vi "MV3D RGBD Get Gig E Device List.vi"(10 "nMaxDeviceCount":u32) -> (0 "pDeviceCount out":u32, 1 "MV3D_RGBD_GigEDEVICE_ByteINFO out":T1(array[cluster]), 2 "MV3D_RGBD_GigEDEVICE_INFO out":T2(array[cluster]), 3 "function return":i32)   [LabVIEW 2015, in "Mv3dRgbdEx.lvlib"]
doc: "MV3D_RGBD_API_Ex MV3D_RGBD_STATUS MV3D_RGBD_GetGigEDeviceList(MV3D_RGBD_GigEDEVICE_INFO* pstGigEDeviceInfos, uint32_t nMaxDeviceCount, uint32_t* pDeviceCount);"
uses:
  <userlib>/Mv3dRgbdEx/Mv3dRgbdEx.lvlib
  <userlib>/Mv3dRgbdEx/Mv3dRgbdEx.dll
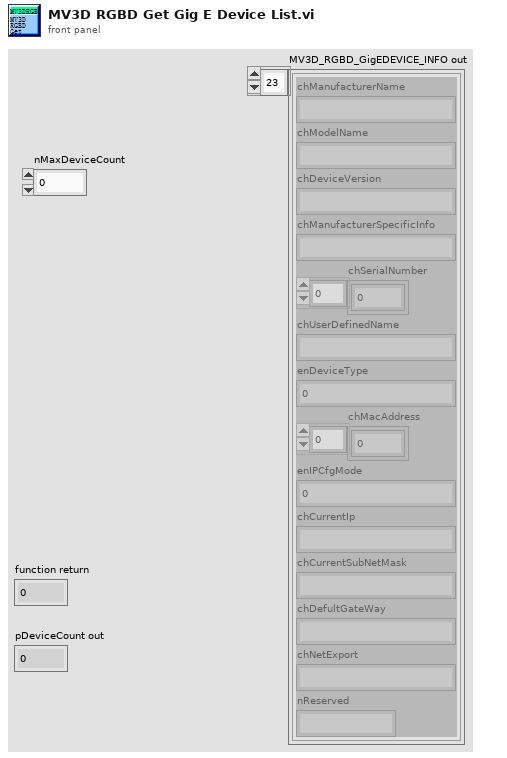
[diagram p1: front panel]
types:
  T1 = cluster{"chManufacturerName[0]":i8, "chManufacturerName[1]":i8, "chManufacturerName[2]":i8, "chManufacturerName[3]":i8, "chManufacturerName[4]":i8, "chManufacturerName[5]":i8, "chManufacturerName[6]":i8, "chManufacturerName[7]":i8, "chManufacturerName[8]":i8, "chManufacturerName[9]":i8, "chManufacturerName[10]":i8, "chManufacturerName[11]":i8, "chManufacturerName[12]":i8, "chManufacturerName[13]":i8, "chManufacturerName[14]":i8, "chManufacturerName[15]":i8, "chManufacturerName[16]":i8, "chManufacturerName[17]":i8, "chManufacturerName[18]":i8, "chManufacturerName[19]":i8, "chManufacturerName[20]":i8, "chManufacturerName[21]":i8, "chManufacturerName[22]":i8, "chManufacturerName[23]":i8, "chManufacturerName[24]":i8, "chManufacturerName[25]":i8, "chManufacturerName[26]":i8, "chManufacturerName[27]":i8, "chManufacturerName[28]":i8, "chManufacturerName[29]":i8, "chManufacturerName[30]":i8, "chManufacturerName[31]":i8, "chModelName[0]":i8, "chModelName[1]":i8, "chModelName[2]":i8, "chModelName[3]":i8, "chModelName[4]":i8, "chModelName[5]":i8, "chModelName[6]":i8, "chModelName[7]":i8, "chModelName[8]":i8, "chModelName[9]":i8, "chModelName[10]":i8, "chModelName[11]":i8, "chModelName[12]":i8, "chModelName[13]":i8, "chModelName[14]":i8, "chModelName[15]":i8, "chModelName[16]":i8, "chModelName[17]":i8, "chModelName[18]":i8, "chModelName[19]":i8, "chModelName[20]":i8, "chModelName[21]":i8, "chModelName[22]":i8, "chModelName[23]":i8, "chModelName[24]":i8, "chModelName[25]":i8, "chModelName[26]":i8, "chModelName[27]":i8, "chModelName[28]":i8, "chModelName[29]":i8, "chModelName[30]":i8, "chModelName[31]":i8, "chDeviceVersion[0]":i8, "chDeviceVersion[1]":i8, "chDeviceVersion[2]":i8, "chDeviceVersion[3]":i8, "chDeviceVersion[4]":i8, "chDeviceVersion[5]":i8, "chDeviceVersion[6]":i8, "chDeviceVersion[7]":i8, "chDeviceVersion[8]":i8, "chDeviceVersion[9]":i8, "chDeviceVersion[10]":i8, "chDeviceVersion[11]":i8, "chDeviceVersion[12]":i8, "chDeviceVersion[13]":i8, "chDeviceVersion[14]":i8, "chDeviceVersion[15]":i8, "chDeviceVersion[16]":i8, "chDeviceVersion[17]":i8, "chDeviceVersion[18]":i8, "chDeviceVersion[19]":i8, "chDeviceVersion[20]":i8, "chDeviceVersion[21]":i8, "chDeviceVersion[22]":i8, "chDeviceVersion[23]":i8, "chDeviceVersion[24]":i8, "chDeviceVersion[25]":i8, "chDeviceVersion[26]":i8, "chDeviceVersion[27]":i8, "chDeviceVersion[28]":i8, "chDeviceVersion[29]":i8, "chDeviceVersion[30]":i8, "chDeviceVersion[31]":i8, "chManufacturerSpecificInfo[0]":i8, "chManufacturerSpecificInfo[1]":i8, "chManufacturerSpecificInfo[2]":i8, "chManufacturerSpecificInfo[3]":i8, "chManufacturerSpecificInfo[4]":i8, "chManufacturerSpecificInfo[5]":i8, "chManufacturerSpecificInfo[6]":i8, "chManufacturerSpecificInfo[7]":i8, "chManufacturerSpecificInfo[8]":i8, "chManufacturerSpecificInfo[9]":i8, "chManufacturerSpecificInfo[10]":i8, "chManufacturerSpecificInfo[11]":i8, "chManufacturerSpecificInfo[12]":i8, "chManufacturerSpecificInfo[13]":i8, "chManufacturerSpecificInfo[14]":i8, "chManufacturerSpecificInfo[15]":i8, "chManufacturerSpecificInfo[16]":i8, "chManufacturerSpecificInfo[17]":i8, "chManufacturerSpecificInfo[18]":i8, "chManufacturerSpecificInfo[19]":i8, "chManufacturerSpecificInfo[20]":i8, "chManufacturerSpecificInfo[21]":i8, "chManufacturerSpecificInfo[22]":i8, "chManufacturerSpecificInfo[23]":i8, "chManufacturerSpecificInfo[24]":i8, "chManufacturerSpecificInfo[25]":i8, "chManufacturerSpecificInfo[26]":i8, "chManufacturerSpecificInfo[27]":i8, "chManufacturerSpecificInfo[28]":i8, "chManufacturerSpecificInfo[29]":i8, "chManufacturerSpecificInfo[30]":i8, "chManufacturerSpecificInfo[31]":i8, "chManufacturerSpecificInfo[32]":i8, "chManufacturerSpecificInfo[33]":i8, "chManufacturerSpecificInfo[34]":i8, "chManufacturerSpecificInfo[35]":i8, "chManufacturerSpecificInfo[36]":i8, "chManufacturerSpecificInfo[37]":i8, "chManufacturerSpecificInfo[38]":i8, "chManufacturerSpecificInfo[39]":i8, "chManufacturerSpecificInfo[40]":i8, "chManufacturerSpecificInfo[41]":i8, "chManufacturerSpecificInfo[42]":i8, "chManufacturerSpecificInfo[43]":i8, "chManufacturerSpecificInfo[44]":i8, "chManufacturerSpecificInfo[45]":i8, "chManufacturerSpecificInfo[46]":i8, "chManufacturerSpecificInfo[47]":i8, "chSerialNumber[0]":i8, "chSerialNumber[1]":i8, "chSerialNumber[2]":i8, "chSerialNumber[3]":i8, "chSerialNumber[4]":i8, "chSerialNumber[5]":i8, "chSerialNumber[6]":i8, "chSerialNumber[7]":i8, "chSerialNumber[8]":i8, "chSerialNumber[9]":i8, "chSerialNumber[10]":i8, "chSerialNumber[11]":i8, "chSerialNumber[12]":i8, "chSerialNumber[13]":i8, "chSerialNumber[14]":i8, "chSerialNumber[15]":i8, "chUserDefinedName[0]":i8, "chUserDefinedName[1]":i8, "chUserDefinedName[2]":i8, "chUserDefinedName[3]":i8, "chUserDefinedName[4]":i8, "chUserDefinedName[5]":i8, "chUserDefinedName[6]":i8, "chUserDefinedName[7]":i8, "chUserDefinedName[8]":i8, "chUserDefinedName[9]":i8, "chUserDefinedName[10]":i8, "chUserDefinedName[11]":i8, "chUserDefinedName[12]":i8, "chUserDefinedName[13]":i8, "chUserDefinedName[14]":i8, "chUserDefinedName[15]":i8, "enDeviceType":i32, "chMacAddress[0]":u8, "chMacAddress[1]":u8, "chMacAddress[2]":u8, "chMacAddress[3]":u8, "chMacAddress[4]":u8, "chMacAddress[5]":u8, "chMacAddress[6]":u8, "chMacAddress[7]":u8, "enIPCfgMode":i32, "chCurrentIp[0]":i8, "chCurrentIp[1]":i8, "chCurrentIp[2]":i8, "chCurrentIp[3]":i8, "chCurrentIp[4]":i8, "chCurrentIp[5]":i8, "chCurrentIp[6]":i8, "chCurrentIp[7]":i8, "chCurrentIp[8]":i8, "chCurrentIp[9]":i8, "chCurrentIp[10]":i8, "chCurrentIp[11]":i8, "chCurrentIp[12]":i8, "chCurrentIp[13]":i8, "chCurrentIp[14]":i8, "chCurrentIp[15]":i8, "chCurrentSubNetMask[0]":i8, "chCurrentSubNetMask[1]":i8, "chCurrentSubNetMask[2]":i8, "chCurrentSubNetMask[3]":i8, "chCurrentSubNetMask[4]":i8, "chCurrentSubNetMask[5]":i8, "chCurrentSubNetMask[6]":i8, "chCurrentSubNetMask[7]":i8, "chCurrentSubNetMask[8]":i8, "chCurrentSubNetMask[9]":i8, "chCurrentSubNetMask[10]":i8, "chCurrentSubNetMask[11]":i8, "chCurrentSubNetMask[12]":i8, "chCurrentSubNetMask[13]":i8, "chCurrentSubNetMask[14]":i8, "chCurrentSubNetMask[15]":i8, "chDefultGateWay[0]":i8, "chDefultGateWay[1]":i8, "chDefultGateWay[2]":i8, "chDefultGateWay[3]":i8, "chDefultGateWay[4]":i8, "chDefultGateWay[5]":i8, "chDefultGateWay[6]":i8, "chDefultGateWay[7]":i8, "chDefultGateWay[8]":i8, "chDefultGateWay[9]":i8, "chDefultGateWay[10]":i8, "chDefultGateWay[11]":i8, "chDefultGateWay[12]":i8, "chDefultGateWay[13]":i8, "chDefultGateWay[14]":i8, "chDefultGateWay[15]":i8, "chNetExport[0]":i8, "chNetExport[1]":i8, "chNetExport[2]":i8, "chNetExport[3]":i8, "chNetExport[4]":i8, "chNetExport[5]":i8, "chNetExport[6]":i8, "chNetExport[7]":i8, "chNetExport[8]":i8, "chNetExport[9]":i8, "chNetExport[10]":i8, "chNetExport[11]":i8, "chNetExport[12]":i8, "chNetExport[13]":i8, "chNetExport[14]":i8, "chNetExport[15]":i8, "nReserved[0]":u8, "nReserved[1]":u8, "nReserved[2]":u8, "nReserved[3]":u8, "nReserved[4]":u8, "nReserved[5]":u8, "nReserved[6]":u8, "nReserved[7]":u8, "nReserved[8]":u8, "nReserved[9]":u8, "nReserved[10]":u8, "nReserved[11]":u8, "nReserved[12]":u8, "nReserved[13]":u8, "nReserved[14]":u8, "nReserved[15]":u8}[]
  T2 = cluster{"chManufacturerName":string, "chModelName":string, "chDeviceVersion":string, "chManufacturerSpecificInfo":string, "chSerialNumber":u8[], "chUserDefinedName":string, "enDeviceType":i32, "chMacAddress":u8[], "enIPCfgMode":i32, "chCurrentIp":string, "chCurrentSubNetMask":string, "chDefultGateWay":string, "chNetExport":string, "nReserved":string}[]
  T3 = cluster{"chManufacturerName[0]":i8, "chManufacturerName[1]":i8, "chManufacturerName[2]":i8, "chManufacturerName[3]":i8, "chManufacturerName[4]":i8, "chManufacturerName[5]":i8, "chManufacturerName[6]":i8, "chManufacturerName[7]":i8, "chManufacturerName[8]":i8, "chManufacturerName[9]":i8, "chManufacturerName[10]":i8, "chManufacturerName[11]":i8, "chManufacturerName[12]":i8, "chManufacturerName[13]":i8, "chManufacturerName[14]":i8, "chManufacturerName[15]":i8, "chManufacturerName[16]":i8, "chManufacturerName[17]":i8, "chManufacturerName[18]":i8, "chManufacturerName[19]":i8, "chManufacturerName[20]":i8, "chManufacturerName[21]":i8, "chManufacturerName[22]":i8, "chManufacturerName[23]":i8, "chManufacturerName[24]":i8, "chManufacturerName[25]":i8, "chManufacturerName[26]":i8, "chManufacturerName[27]":i8, "chManufacturerName[28]":i8, "chManufacturerName[29]":i8, "chManufacturerName[30]":i8, "chManufacturerName[31]":i8, "chModelName[0]":i8, "chModelName[1]":i8, "chModelName[2]":i8, "chModelName[3]":i8, "chModelName[4]":i8, "chModelName[5]":i8, "chModelName[6]":i8, "chModelName[7]":i8, "chModelName[8]":i8, "chModelName[9]":i8, "chModelName[10]":i8, "chModelName[11]":i8, "chModelName[12]":i8, "chModelName[13]":i8, "chModelName[14]":i8, "chModelName[15]":i8, "chModelName[16]":i8, "chModelName[17]":i8, "chModelName[18]":i8, "chModelName[19]":i8, "chModelName[20]":i8, "chModelName[21]":i8, "chModelName[22]":i8, "chModelName[23]":i8, "chModelName[24]":i8, "chModelName[25]":i8, "chModelName[26]":i8, "chModelName[27]":i8, "chModelName[28]":i8, "chModelName[29]":i8, "chModelName[30]":i8, "chModelName[31]":i8, "chDeviceVersion[0]":i8, "chDeviceVersion[1]":i8, "chDeviceVersion[2]":i8, "chDeviceVersion[3]":i8, "chDeviceVersion[4]":i8, "chDeviceVersion[5]":i8, "chDeviceVersion[6]":i8, "chDeviceVersion[7]":i8, "chDeviceVersion[8]":i8, "chDeviceVersion[9]":i8, "chDeviceVersion[10]":i8, "chDeviceVersion[11]":i8, "chDeviceVersion[12]":i8, "chDeviceVersion[13]":i8, "chDeviceVersion[14]":i8, "chDeviceVersion[15]":i8, "chDeviceVersion[16]":i8, "chDeviceVersion[17]":i8, "chDeviceVersion[18]":i8, "chDeviceVersion[19]":i8, "chDeviceVersion[20]":i8, "chDeviceVersion[21]":i8, "chDeviceVersion[22]":i8, "chDeviceVersion[23]":i8, "chDeviceVersion[24]":i8, "chDeviceVersion[25]":i8, "chDeviceVersion[26]":i8, "chDeviceVersion[27]":i8, "chDeviceVersion[28]":i8, "chDeviceVersion[29]":i8, "chDeviceVersion[30]":i8, "chDeviceVersion[31]":i8, "chManufacturerSpecificInfo[0]":i8, "chManufacturerSpecificInfo[1]":i8, "chManufacturerSpecificInfo[2]":i8, "chManufacturerSpecificInfo[3]":i8, "chManufacturerSpecificInfo[4]":i8, "chManufacturerSpecificInfo[5]":i8, "chManufacturerSpecificInfo[6]":i8, "chManufacturerSpecificInfo[7]":i8, "chManufacturerSpecificInfo[8]":i8, "chManufacturerSpecificInfo[9]":i8, "chManufacturerSpecificInfo[10]":i8, "chManufacturerSpecificInfo[11]":i8, "chManufacturerSpecificInfo[12]":i8, "chManufacturerSpecificInfo[13]":i8, "chManufacturerSpecificInfo[14]":i8, "chManufacturerSpecificInfo[15]":i8, "chManufacturerSpecificInfo[16]":i8, "chManufacturerSpecificInfo[17]":i8, "chManufacturerSpecificInfo[18]":i8, "chManufacturerSpecificInfo[19]":i8, "chManufacturerSpecificInfo[20]":i8, "chManufacturerSpecificInfo[21]":i8, "chManufacturerSpecificInfo[22]":i8, "chManufacturerSpecificInfo[23]":i8, "chManufacturerSpecificInfo[24]":i8, "chManufacturerSpecificInfo[25]":i8, "chManufacturerSpecificInfo[26]":i8, "chManufacturerSpecificInfo[27]":i8, "chManufacturerSpecificInfo[28]":i8, "chManufacturerSpecificInfo[29]":i8, "chManufacturerSpecificInfo[30]":i8, "chManufacturerSpecificInfo[31]":i8, "chManufacturerSpecificInfo[32]":i8, "chManufacturerSpecificInfo[33]":i8, "chManufacturerSpecificInfo[34]":i8, "chManufacturerSpecificInfo[35]":i8, "chManufacturerSpecificInfo[36]":i8, "chManufacturerSpecificInfo[37]":i8, "chManufacturerSpecificInfo[38]":i8, "chManufacturerSpecificInfo[39]":i8, "chManufacturerSpecificInfo[40]":i8, "chManufacturerSpecificInfo[41]":i8, "chManufacturerSpecificInfo[42]":i8, "chManufacturerSpecificInfo[43]":i8, "chManufacturerSpecificInfo[44]":i8, "chManufacturerSpecificInfo[45]":i8, "chManufacturerSpecificInfo[46]":i8, "chManufacturerSpecificInfo[47]":i8, "chSerialNumber[0]":i8, "chSerialNumber[1]":i8, "chSerialNumber[2]":i8, "chSerialNumber[3]":i8, "chSerialNumber[4]":i8, "chSerialNumber[5]":i8, "chSerialNumber[6]":i8, "chSerialNumber[7]":i8, "chSerialNumber[8]":i8, "chSerialNumber[9]":i8, "chSerialNumber[10]":i8, "chSerialNumber[11]":i8, "chSerialNumber[12]":i8, "chSerialNumber[13]":i8, "chSerialNumber[14]":i8, "chSerialNumber[15]":i8, "chUserDefinedName[0]":i8, "chUserDefinedName[1]":i8, "chUserDefinedName[2]":i8, "chUserDefinedName[3]":i8, "chUserDefinedName[4]":i8, "chUserDefinedName[5]":i8, "chUserDefinedName[6]":i8, "chUserDefinedName[7]":i8, "chUserDefinedName[8]":i8, "chUserDefinedName[9]":i8, "chUserDefinedName[10]":i8, "chUserDefinedName[11]":i8, "chUserDefinedName[12]":i8, "chUserDefinedName[13]":i8, "chUserDefinedName[14]":i8, "chUserDefinedName[15]":i8, "enDeviceType":i32, "chMacAddress[0]":u8, "chMacAddress[1]":u8, "chMacAddress[2]":u8, "chMacAddress[3]":u8, "chMacAddress[4]":u8, "chMacAddress[5]":u8, "chMacAddress[6]":u8, "chMacAddress[7]":u8, "enIPCfgMode":i32, "chCurrentIp[0]":i8, "chCurrentIp[1]":i8, "chCurrentIp[2]":i8, "chCurrentIp[3]":i8, "chCurrentIp[4]":i8, "chCurrentIp[5]":i8, "chCurrentIp[6]":i8, "chCurrentIp[7]":i8, "chCurrentIp[8]":i8, "chCurrentIp[9]":i8, "chCurrentIp[10]":i8, "chCurrentIp[11]":i8, "chCurrentIp[12]":i8, "chCurrentIp[13]":i8, "chCurrentIp[14]":i8, "chCurrentIp[15]":i8, "chCurrentSubNetMask[0]":i8, "chCurrentSubNetMask[1]":i8, "chCurrentSubNetMask[2]":i8, "chCurrentSubNetMask[3]":i8, "chCurrentSubNetMask[4]":i8, "chCurrentSubNetMask[5]":i8, "chCurrentSubNetMask[6]":i8, "chCurrentSubNetMask[7]":i8, "chCurrentSubNetMask[8]":i8, "chCurrentSubNetMask[9]":i8, "chCurrentSubNetMask[10]":i8, "chCurrentSubNetMask[11]":i8, "chCurrentSubNetMask[12]":i8, "chCurrentSubNetMask[13]":i8, "chCurrentSubNetMask[14]":i8, "chCurrentSubNetMask[15]":i8, "chDefultGateWay[0]":i8, "chDefultGateWay[1]":i8, "chDefultGateWay[2]":i8, "chDefultGateWay[3]":i8, "chDefultGateWay[4]":i8, "chDefultGateWay[5]":i8, "chDefultGateWay[6]":i8, "chDefultGateWay[7]":i8, "chDefultGateWay[8]":i8, "chDefultGateWay[9]":i8, "chDefultGateWay[10]":i8, "chDefultGateWay[11]":i8, "chDefultGateWay[12]":i8, "chDefultGateWay[13]":i8, "chDefultGateWay[14]":i8, "chDefultGateWay[15]":i8, "chNetExport[0]":i8, "chNetExport[1]":i8, "chNetExport[2]":i8, "chNetExport[3]":i8, "chNetExport[4]":i8, "chNetExport[5]":i8, "chNetExport[6]":i8, "chNetExport[7]":i8, "chNetExport[8]":i8, "chNetExport[9]":i8, "chNetExport[10]":i8, "chNetExport[11]":i8, "chNetExport[12]":i8, "chNetExport[13]":i8, "chNetExport[14]":i8, "chNetExport[15]":i8, "nReserved[0]":u8, "nReserved[1]":u8, "nReserved[2]":u8, "nReserved[3]":u8, "nReserved[4]":u8, "nReserved[5]":u8, "nReserved[6]":u8, "nReserved[7]":u8, "nReserved[8]":u8, "nReserved[9]":u8, "nReserved[10]":u8, "nReserved[11]":u8, "nReserved[12]":u8, "nReserved[13]":u8, "nReserved[14]":u8, "nReserved[15]":u8}
  T4 = cluster{"chManufacturerName":string, "chModelName":string, "chDeviceVersion":string, "chManufacturerSpecificInfo":string, "chSerialNumber":u8[], "chUserDefinedName":string, "enDeviceType":i32, "chMacAddress":u8[], "enIPCfgMode":i32, "chCurrentIp":string, "chCurrentSubNetMask":string, "chDefultGateWay":string, "chNetExport":string, "nReserved":string}
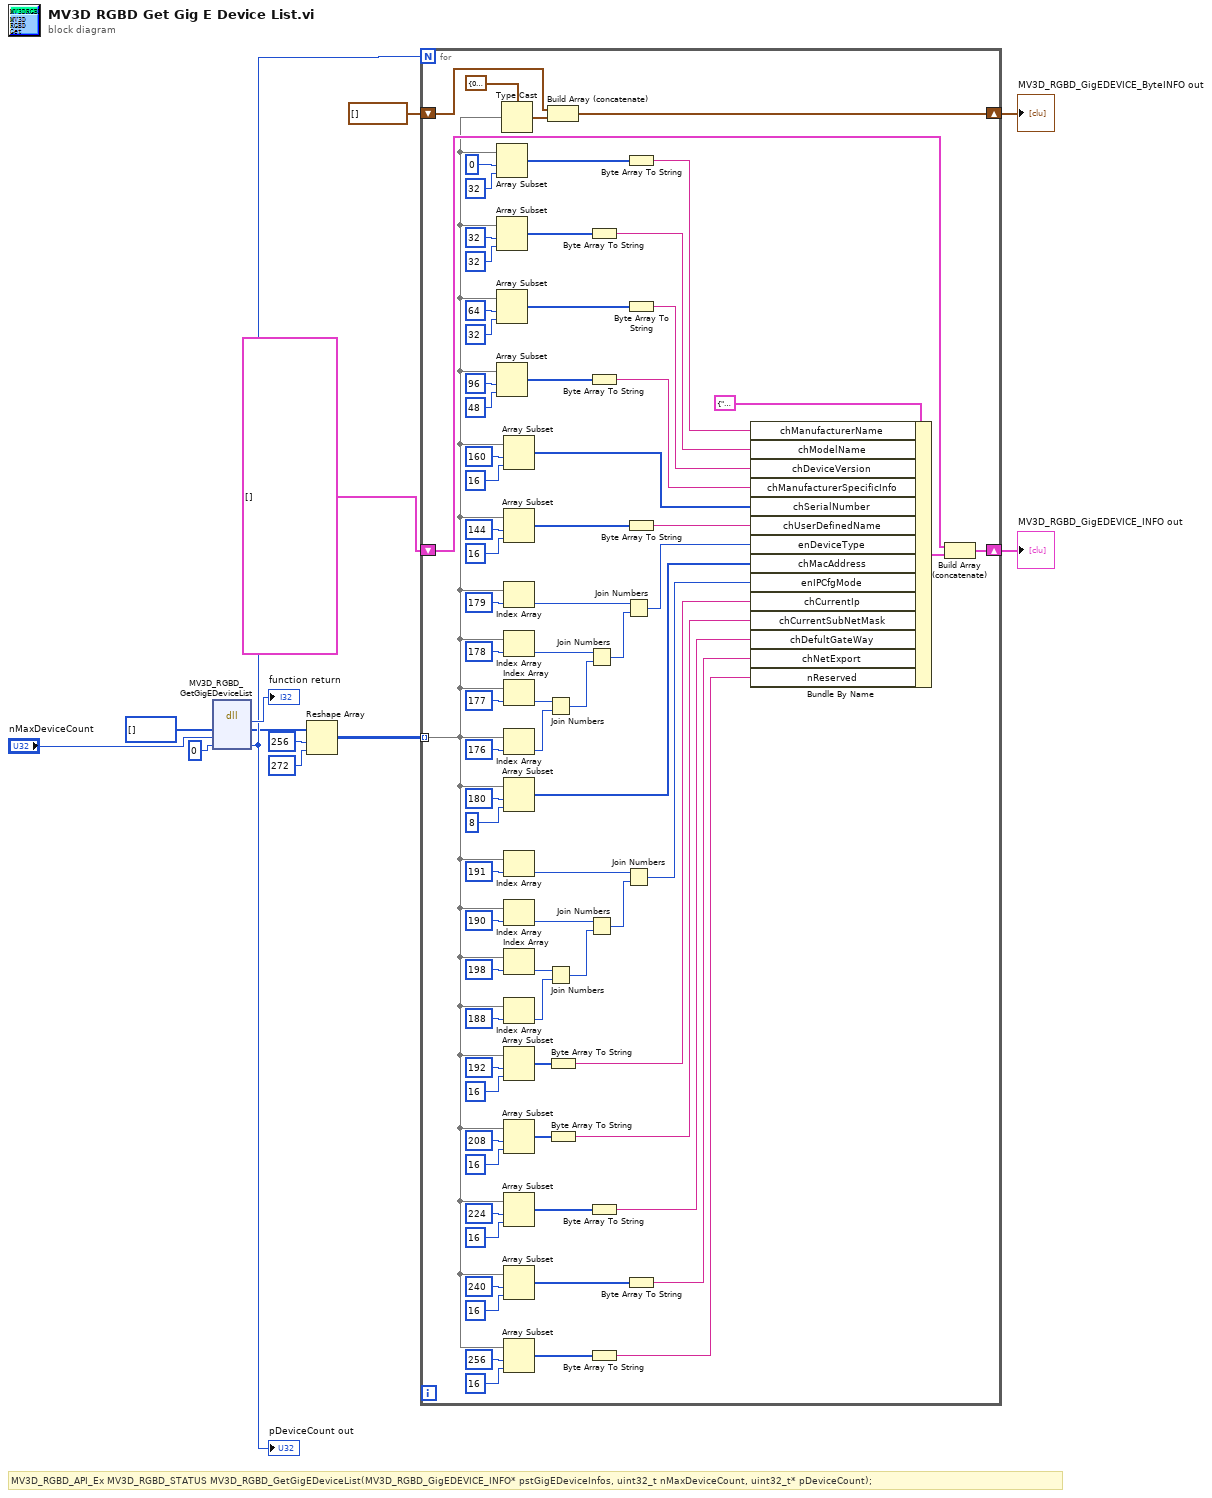
[diagram p0: block diagram]
diagram:
  # "MV3D_RGBD_API_Ex MV3D_RGBD_STATUS MV3D_RGBD_GetGigEDeviceList(MV3D_RGBD_GigEDEVICE_INFO* pstGigEDeviceInfos, uint32_t nMaxDeviceCount, uint32_t* pDeviceCount);"
  n1 = dll-call lib="C:/Program Files (x86)/National Instruments/LabVIEW 2015/user.lib/Mv3dRgbdEx/Mv3dRgbdEx.*" fn="MV3D_RGBD_GetGigEDeviceList"("pstGigEDeviceInfos"=u8[] [] ("pstGigEDeviceInfos 4"), "nMaxDeviceCount"="nMaxDeviceCount", "pDeviceCount"=u32 0) -> ("返回类型"=→"function return":i32, "pstGigEDeviceInfos"=w8:u8[], "pDeviceCount"=w9:u32)  [unwired: 4 in, 2 out]
  "pDeviceCount out" <- w9
  n2 = Reshape Array(w8, 256 ("维数大小"), 272 ("维数大小")) -> (w5:u8[][])
  n3 = for {
    N: w9 -> [_]
    shift-right: [w46] -> w3
    shift-left: T2 [] -> [w19]
    tunnel: w5 -> [w17] mode=indexing
    shift-right: [w16] -> w2
    shift-left: T1 [] ("*(类型 *) &x") -> [w14]
    n4 = Array Subset(array=w17, index=0 ("索引"), length=32 ("长度")) -> (w88:u8[])
    n5 = Array Subset(array=w17, index=32 ("索引"), length=32 ("长度")) -> (w85:u8[])
    n6 = Array Subset(array=w17, index=64 ("索引"), length=32 ("长度")) -> (w78:u8[])
    n7 = Array Subset(array=w17, index=96 ("索引"), length=48 ("长度")) -> (w82:u8[])
    n8 = Type Cast(type=T3 {"chManufacturerName[0]"=0, "chManufacturerName[1]"=0, "chManufacturerName[2]"=0, "chManufacturerName[3]"=0, "chManufacturerName[4]"=0, "chManufacturerName[5]"=0, "chManufacturerName[6]"=0, "chManufacturerName[7]"=0, "chManufacturerName[8]"=0, "chManufacturerName[9]"=0, "chManufacturerName[10]"=0, "chManufacturerName[11]"=0, "chManufacturerName[12]"=0, "chManufacturerName[13]"=0, "chManufacturerName[14]"=0, "chManufacturerName[15]"=0, "chManufacturerName[16]"=0, "chManufacturerName[17]"=0, "chManufacturerName[18]"=0, "chManufacturerName[19]"=0, "chManufacturerName[20]"=0, "chManufacturerName[21]"=0, "chManufacturerName[22]"=0, "chManufacturerName[23]"=0, "chManufacturerName[24]"=0, "chManufacturerName[25]"=0, "chManufacturerName[26]"=0, "chManufacturerName[27]"=0, "chManufacturerName[28]"=0, "chManufacturerName[29]"=0, "chManufacturerName[30]"=0, "chManufacturerName[31]"=0, "chModelName[0]"=0, "chModelName[1]"=0, "chModelName[2]"=0, "chModelName[3]"=0, "chModelName[4]"=0, "chModelName[5]"=0, "chModelName[6]"=0, "chModelName[7]"=0, "chModelName[8]"=0, "chModelName[9]"=0, "chModelName[10]"=0, "chModelName[11]"=0, "chModelName[12]"=0, "chModelName[13]"=0, "chModelName[14]"=0, "chModelName[15]"=0, "chModelName[16]"=0, "chModelName[17]"=0, "chModelName[18]"=0, "chModelName[19]"=0, "chModelName[20]"=0, "chModelName[21]"=0, "chModelName[22]"=0, "chModelName[23]"=0, "chModelName[24]"=0, "chModelName[25]"=0, "chModelName[26]"=0, "chModelName[27]"=0, "chModelName[28]"=0, "chModelName[29]"=0, "chModelName[30]"=0, "chModelName[31]"=0, "chDeviceVersion[0]"=0, "chDeviceVersion[1]"=0, "chDeviceVersion[2]"=0, "chDeviceVersion[3]"=0, "chDeviceVersion[4]"=0, "chDeviceVersion[5]"=0, "chDeviceVersion[6]"=0, "chDeviceVersion[7]"=0, "chDeviceVersion[8]"=0, "chDeviceVersion[9]"=0, "chDeviceVersion[10]"=0, "chDeviceVersion[11]"=0, "chDeviceVersion[12]"=0, "chDeviceVersion[13]"=0, "chDeviceVersion[14]"=0, "chDeviceVersion[15]"=0, "chDeviceVersion[16]"=0, "chDeviceVersion[17]"=0, "chDeviceVersion[18]"=0, "chDeviceVersion[19]"=0, "chDeviceVersion[20]"=0, "chDeviceVersion[21]"=0, "chDeviceVersion[22]"=0, "chDeviceVersion[23]"=0, "chDeviceVersion[24]"=0, "chDeviceVersion[25]"=0, "chDeviceVersion[26]"=0, "chDeviceVersion[27]"=0, "chDeviceVersion[28]"=0, "chDeviceVersion[29]"=0, "chDeviceVersion[30]"=0, "chDeviceVersion[31]"=0, "chManufacturerSpecificInfo[0]"=0, "chManufacturerSpecificInfo[1]"=0, "chManufacturerSpecificInfo[2]"=0, "chManufacturerSpecificInfo[3]"=0, "chManufacturerSpecificInfo[4]"=0, "chManufacturerSpecificInfo[5]"=0, "chManufacturerSpecificInfo[6]"=0, "chManufacturerSpecificInfo[7]"=0, "chManufacturerSpecificInfo[8]"=0, "chManufacturerSpecificInfo[9]"=0, "chManufacturerSpecificInfo[10]"=0, "chManufacturerSpecificInfo[11]"=0, "chManufacturerSpecificInfo[12]"=0, "chManufacturerSpecificInfo[13]"=0, "chManufacturerSpecificInfo[14]"=0, "chManufacturerSpecificInfo[15]"=0, "chManufacturerSpecificInfo[16]"=0, "chManufacturerSpecificInfo[17]"=0, "chManufacturerSpecificInfo[18]"=0, "chManufacturerSpecificInfo[19]"=0, "chManufacturerSpecificInfo[20]"=0, "chManufacturerSpecificInfo[21]"=0, "chManufacturerSpecificInfo[22]"=0, "chManufacturerSpecificInfo[23]"=0, "chManufacturerSpecificInfo[24]"=0, "chManufacturerSpecificInfo[25]"=0, "chManufacturerSpecificInfo[26]"=0, "chManufacturerSpecificInfo[27]"=0, "chManufacturerSpecificInfo[28]"=0, "chManufacturerSpecificInfo[29]"=0, "chManufacturerSpecificInfo[30]"=0, "chManufacturerSpecificInfo[31]"=0, "chManufacturerSpecificInfo[32]"=0, "chManufacturerSpecificInfo[33]"=0, "chManufacturerSpecificInfo[34]"=0, "chManufacturerSpecificInfo[35]"=0, "chManufacturerSpecificInfo[36]"=0, "chManufacturerSpecificInfo[37]"=0, "chManufacturerSpecificInfo[38]"=0, "chManufacturerSpecificInfo[39]"=0, "chManufacturerSpecificInfo[40]"=0, "chManufacturerSpecificInfo[41]"=0, "chManufacturerSpecificInfo[42]"=0, "chManufacturerSpecificInfo[43]"=0, "chManufacturerSpecificInfo[44]"=0, "chManufacturerSpecificInfo[45]"=0, "chManufacturerSpecificInfo[46]"=0, "chManufacturerSpecificInfo[47]"=0, "chSerialNumber[0]"=0, "chSerialNumber[1]"=0, "chSerialNumber[2]"=0, "chSerialNumber[3]"=0, "chSerialNumber[4]"=0, "chSerialNumber[5]"=0, "chSerialNumber[6]"=0, "chSerialNumber[7]"=0, "chSerialNumber[8]"=0, "chSerialNumber[9]"=0, "chSerialNumber[10]"=0, "chSerialNumber[11]"=0, "chSerialNumber[12]"=0, "chSerialNumber[13]"=0, "chSerialNumber[14]"=0, "chSerialNumber[15]"=0, "chUserDefinedName[0]"=0, "chUserDefinedName[1]"=0, "chUserDefinedName[2]"=0, "chUserDefinedName[3]"=0, "chUserDefinedName[4]"=0, "chUserDefinedName[5]"=0, "chUserDefinedName[6]"=0, "chUserDefinedName[7]"=0, "chUserDefinedName[8]"=0, "chUserDefinedName[9]"=0, "chUserDefinedName[10]"=0, "chUserDefinedName[11]"=0, "chUserDefinedName[12]"=0, "chUserDefinedName[13]"=0, "chUserDefinedName[14]"=0, "chUserDefinedName[15]"=0, "enDeviceType"=0, "chMacAddress[0]"=0, "chMacAddress[1]"=0, "chMacAddress[2]"=0, "chMacAddress[3]"=0, "chMacAddress[4]"=0, "chMacAddress[5]"=0, "chMacAddress[6]"=0, "chMacAddress[7]"=0, "enIPCfgMode"=0, "chCurrentIp[0]"=0, "chCurrentIp[1]"=0, "chCurrentIp[2]"=0, "chCurrentIp[3]"=0, "chCurrentIp[4]"=0, "chCurrentIp[5]"=0, "chCurrentIp[6]"=0, "chCurrentIp[7]"=0, "chCurrentIp[8]"=0, "chCurrentIp[9]"=0, "chCurrentIp[10]"=0, "chCurrentIp[11]"=0, "chCurrentIp[12]"=0, "chCurrentIp[13]"=0, "chCurrentIp[14]"=0, "chCurrentIp[15]"=0, "chCurrentSubNetMask[0]"=0, "chCurrentSubNetMask[1]"=0, "chCurrentSubNetMask[2]"=0, "chCurrentSubNetMask[3]"=0, "chCurrentSubNetMask[4]"=0, "chCurrentSubNetMask[5]"=0, "chCurrentSubNetMask[6]"=0, "chCurrentSubNetMask[7]"=0, "chCurrentSubNetMask[8]"=0, "chCurrentSubNetMask[9]"=0, "chCurrentSubNetMask[10]"=0, "chCurrentSubNetMask[11]"=0, "chCurrentSubNetMask[12]"=0, "chCurrentSubNetMask[13]"=0, "chCurrentSubNetMask[14]"=0, "chCurrentSubNetMask[15]"=0, "chDefultGateWay[0]"=0, "chDefultGateWay[1]"=0, "chDefultGateWay[2]"=0, "chDefultGateWay[3]"=0, "chDefultGateWay[4]"=0, "chDefultGateWay[5]"=0, "chDefultGateWay[6]"=0, "chDefultGateWay[7]"=0, "chDefultGateWay[8]"=0, "chDefultGateWay[9]"=0, "chDefultGateWay[10]"=0, "chDefultGateWay[11]"=0, "chDefultGateWay[12]"=0, "chDefultGateWay[13]"=0, "chDefultGateWay[14]"=0, "chDefultGateWay[15]"=0, "chNetExport[0]"=0, "chNetExport[1]"=0, "chNetExport[2]"=0, "chNetExport[3]"=0, "chNetExport[4]"=0, "chNetExport[5]"=0, "chNetExport[6]"=0, "chNetExport[7]"=0, "chNetExport[8]"=0, "chNetExport[9]"=0, "chNetExport[10]"=0, "chNetExport[11]"=0, "chNetExport[12]"=0, "chNetExport[13]"=0, "chNetExport[14]"=0, "chNetExport[15]"=0, "nReserved[0]"=0, "nReserved[1]"=0, "nReserved[2]"=0, "nReserved[3]"=0, "nReserved[4]"=0, "nReserved[5]"=0, "nReserved[6]"=0, "nReserved[7]"=0, "nReserved[8]"=0, "nReserved[9]"=0, "nReserved[10]"=0, "nReserved[11]"=0, "nReserved[12]"=0, "nReserved[13]"=0, "nReserved[14]"=0, "nReserved[15]"=0} ("pstGigeDeviceInfo out"), x=w17) -> (*(type *) &x=w15:T3)
    n9 = Array Subset(array=w17, index=160 ("索引"), length=16 ("长度")) -> (w28:u8[])
    n10 = Array Subset(array=w17, index=144 ("索引"), length=16 ("长度")) -> (w79:u8[])
    n11 = Index Array(array=w17, index=179 ("索引")) -> (element=w21:u8)
    n12 = Index Array(array=w17, index=178 ("索引")) -> (element=w22:u8)
    n13 = Index Array(array=w17, index=177 ("索引")) -> (element=w24:u8)
    n14 = Index Array(array=w17, index=176 ("索引")) -> (element=w25:u8)
    n15 = Array Subset(array=w17, index=180 ("索引"), length=8 ("长度")) -> (w26:u8[])
    n16 = Index Array(array=w17, index=191 ("索引")) -> (element=w39:u8)
    n17 = Index Array(array=w17, index=190 ("索引")) -> (element=w37:u8)
    n18 = Index Array(array=w17, index=198 ("索引")) -> (element=w35:u8)
    n19 = Index Array(array=w17, index=188 ("索引")) -> (element=w30:u8)
    n20 = Array Subset(array=w17, index=192 ("索引"), length=16 ("长度")) -> (w72:u8[])
    n21 = Array Subset(array=w17, index=208 ("索引"), length=16 ("长度")) -> (w70:u8[])
    n22 = Array Subset(array=w17, index=224 ("索引"), length=16 ("长度")) -> (w68:u8[])
    n23 = Array Subset(array=w17, index=240 ("索引"), length=16 ("长度")) -> (w66:u8[])
    n24 = Array Subset(array=w17, index=256 ("索引"), length=16 ("长度")) -> (w64:u8[])
    n25 = Join Numbers(hi=w24, lo=w25) -> ((hi.lo)=w23:u16)
    n26 = Join Numbers(hi=w35, lo=w30) -> ((hi.lo)=w34:u16)
    n27 = Build Array (concatenate)(w14, w15) -> (w16:T1)
    n28 = Byte Array To String(unsigned byte array=w72) -> (string=w51:string)
    n29 = Byte Array To String(unsigned byte array=w70) -> (string=w50:string)
    n30 = Join Numbers(hi=w22, lo=w23) -> ((hi.lo)=w20:u32)
    n31 = Join Numbers(hi=w37, lo=w34) -> ((hi.lo)=w33:u32)
    n32 = Byte Array To String(unsigned byte array=w85) -> (string=w55:string)
    n33 = Byte Array To String(unsigned byte array=w82) -> (string=w53:string)
    n34 = Byte Array To String(unsigned byte array=w68) -> (string=w49:string)
    n35 = Byte Array To String(unsigned byte array=w64) -> (string=w47:string)
    n36 = Join Numbers(hi=w21, lo=w20) -> ((hi.lo)=w41:u64)
    n37 = Join Numbers(hi=w39, lo=w33) -> ((hi.lo)=w32:u64)
    n38 = Byte Array To String(unsigned byte array=w88) -> (string=w56:string)
    n39 = Byte Array To String(unsigned byte array=w78) -> (string=w54:string)
    n40 = Byte Array To String(unsigned byte array=w79) -> (string=w52:string)
    n41 = Byte Array To String(unsigned byte array=w66) -> (string=w48:string)
    n42 = Bundle By Name(cluster=T4 {"chManufacturerName"="Hikrobot\u0000\u0000\u0000\u0000\u0000\u0000\u0000\u0000\u0000\u0000\u0000\u0000\u0000\u0000\u0000\u0000\u0000\u0000\u0000\u0000\u0000\u0000\u0000\u0000", "chModelName"="MV-DP2307-01H\u0000\u0000\u0000\u0000\u0000\u0000\u0000\u0000\u0000\u0000\u0000\u0000\u0000\u0000\u0000\u0000\u0000\u0000\u0000", "chDeviceVersion"="V1.2.1 220326 783627\u0000\u0000\u0000\u0000\u0000\u0000\u0000\u0000\u0000\u0000\u0000\u0000", "chManufacturerSpecificInfo"="Hikrobot\u0000\u0000\u0000\u0000\u0000\u0000\u0000\u0000\u0000\u0000\u0000\u0000\u0000\u0000\u0000\u0000\u0000\u0000\u0000\u0000\u0000\u0000\u0000\u0000\u0000\u0000\u0000\u0000\u0000\u0000\u0000\u0000\u0000\u0000\u0000\u0000\u0000\u0000\u0000\u0000", "chSerialNumber"=[], "chUserDefinedName"="00201201207\u0000\u0000\u0000\u0000\u0000", "enDeviceType"=0, "chMacAddress"=[], "enIPCfgMode"=0, "chCurrentIp"="10.108.163.244\u0000\u0000", "chCurrentSubNetMask"="255.255.255.0\u0000\u0000\u0000", "chDefultGateWay"="10.108.163.254\u0000\u0000", "chNetExport"="10.108.163.123\u0000\u0000", "nReserved"="\u0000\u0000\u0000\u0000\u0000\u0000\u0000\u0000\u0000\u0000\u0000\u0000\u0000\u0000\u0000\u0000"} ("MV3D_RGBD_GigEDEVICE_INFO"), "chManufacturerName"=w56, "chModelName"=w55, "chDeviceVersion"=w54, "chManufacturerSpecificInfo"=w53, "chSerialNumber"=w28, "chUserDefinedName"=w52, "enDeviceType"=w41, "chMacAddress"=w26, "enIPCfgMode"=w32, "chCurrentIp"=w51, "chCurrentSubNetMask"=w50, "chDefultGateWay"=w49, "chNetExport"=w48, "nReserved"=w47) -> (w27:T4)
    n43 = Build Array (concatenate)(w19, w27) -> (w46:T2)
  }
  "MV3D_RGBD_GigEDEVICE_INFO out" <- w3
  "MV3D_RGBD_GigEDEVICE_ByteINFO out" <- w2
